vi "PID Autotuning.vi"(4 "autotune? (F)":bool, 5 "autotuning parameters":T2={"controller type"=1, "relay cycles"=3, "relay amplitude"=1.0, "control specification"=2, "PV noise level"=0.1} {"PV noise level" format="%.2f"; "control specification" items=["normal", "fast", "slow"]; "relay amplitude" format="%.2f"; "controller type" items=["PID", "PI", "P"]}, 6 "reinitialize? (F)":bool, 7 "output range":cluster{"output high":dbl, "output low":dbl}={"output high"=100.0, "output low"=-100.0} {"output low" format="%.2f"; "output high" format="%.2f"}, 8 "dt (s)":dbl=-1.0 format="%.3f", 9 "PID gains":T1={"proportional gain (Kc)"=1.0, "integral time (Ti, min)"=0.01, "derivative time (Td, min)"=0.0} {"derivative time (Td, min)" format="%.3f"; "integral time (Ti, min)" format="%.3f"; "proportional gain (Kc)" format="%.3f"}, 10 "process variable":dbl format="%.2f", 11 "setpoint":dbl format="%.2f") -> (0 "dt out (s)":dbl format="%.3f", 1 "PID gains out":T1={"proportional gain (Kc)"=1.0, "integral time (Ti, min)"=0.01, "derivative time (Td, min)"=0.0} {"derivative time (Td, min)" format="%.3f"; "integral time (Ti, min)" format="%.3f"; "proportional gain (Kc)" format="%.3f"}, 2 "tuning completed?":bool, 3 "output":dbl format="%.2f")   [LabVIEW 2017, in "NI_PID_autopid.lvlib"]
doc: "Includes the Autotuning Wizard in addition to the basic PID algorithm. You can use this VI instead of the PID VI, which implements a basic PID algorithm. Use the additional inputs and output of this VI to set autotuning parameters, invoke the Autotuning Wizard, and update the PID gains."
uses:
  <vilib>/addons/control/pid/NI_PID_autopid.lvlib
  <vilib>/addons/control/pid/NI_PID_pid.lvlib
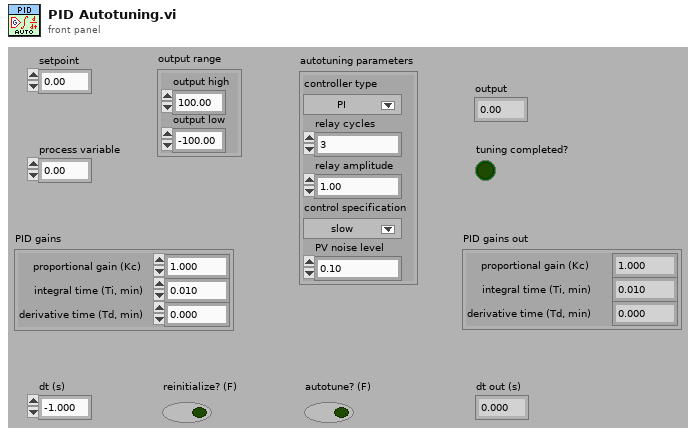
[diagram p1: front panel]
types:
  T1 = cluster{"proportional gain (Kc)":dbl, "integral time (Ti, min)":dbl, "derivative time (Td, min)":dbl}
  T2 = cluster{"controller type":u16, "relay cycles":i32, "relay amplitude":dbl, "control specification":u16, "PV noise level":dbl}
  T3 = enum16{"Normal", "Start", "Check params", "Check noise", "Start noise est.", "Re-estimate noise", "Begin autotune", "Autotuning", "New parameters", ""}
  T4 = cluster{"process variable":dbl, "setpoint out":dbl, "output":dbl}
  T5 = cluster{"Controller Type":u16, "# of cycles to avg":i32, "Relay amplitude":dbl, "Control design  ":u16, "Noise level":dbl}
  T6 = cluster{"Kc":dbl, "Ti (min)":dbl, "Td (min)":dbl}
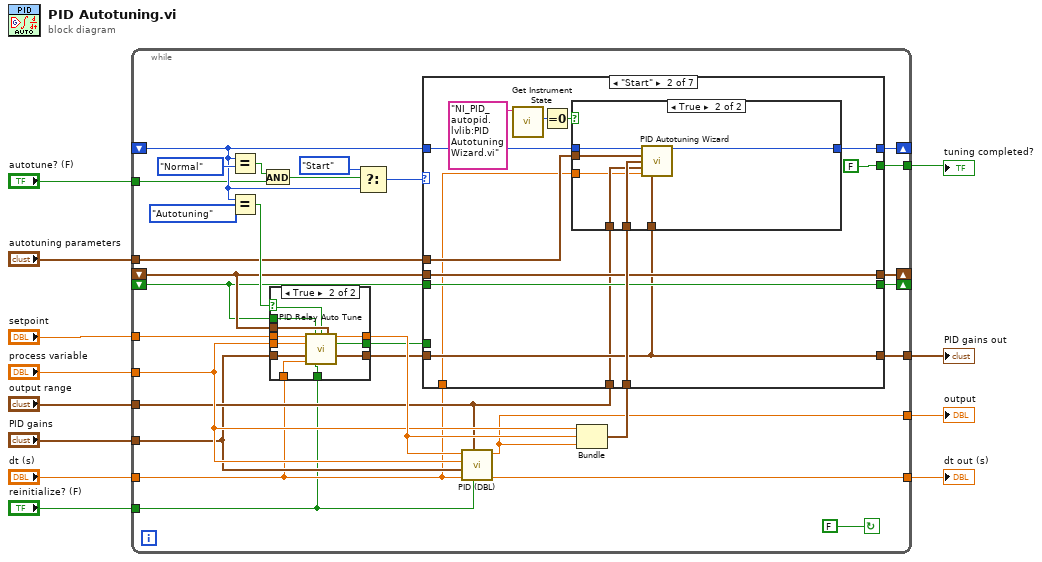
[diagram p0: block diagram]
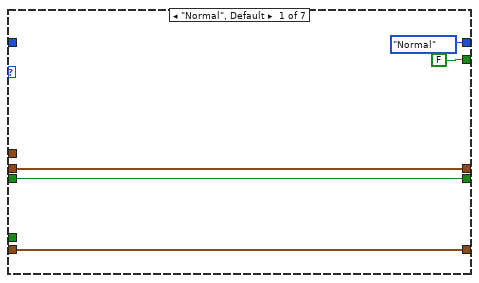
[diagram p2: hidden frame]
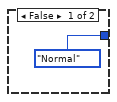
[diagram p3: hidden frame]
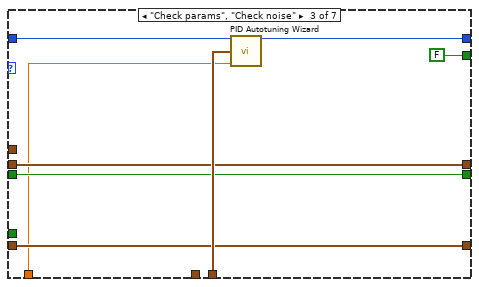
[diagram p4: hidden frame]
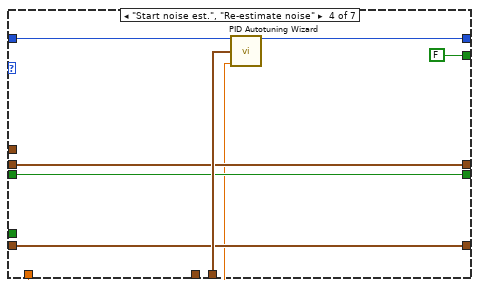
[diagram p5: hidden frame]
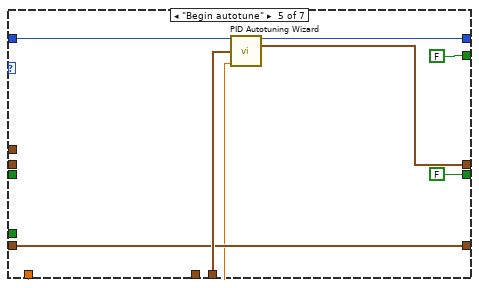
[diagram p6: hidden frame]
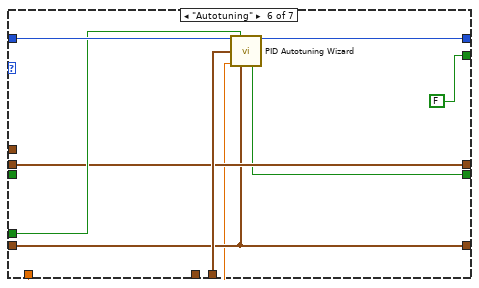
[diagram p7: hidden frame]
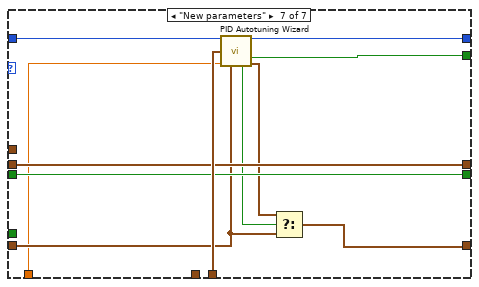
[diagram p8: hidden frame]
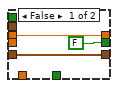
[diagram p9: hidden frame]
diagram:
  n1 = while {
    shift-left: _ -> [w33]
    shift-right: [w32] -> _
    shift-left: _ -> [w34]
    shift-right: [w35] -> _
    shift-left: _ -> [w25]
    shift-right: [w42] -> _
    tunnel: "setpoint" -> [w24]
    tunnel: "process variable" -> [w23]
    tunnel: "output range" -> [w22]
    tunnel: "PID gains" -> [w21]
    tunnel: "dt (s)" -> [w20]
    tunnel: "reinitialize? (F)" -> [w19]
    tunnel: "autotune? (F)" -> [w18]
    tunnel: "autotuning parameters" -> [w17]
    tunnel: [w16] -> w4
    tunnel: [w15] -> w3
    tunnel: [w14] -> w2
    tunnel: [w13] -> w1
    stop <- FALSE continue-if-true
    n2 = Equal?(x=w25, y=T3."Normal" ("states")) -> (x = y?=w31:bool)
    n3 = Equal?(x=w25, y=T3."Autotuning" ("states")) -> (x = y?=w40:bool)
    n4 = And(x=w31, y=w18) -> (x .and. y?=w39:bool)
    n5 = case shown="True" w40 {
      selector: w40 -> [_ w116]
      tunnel: [w115 w117] -> w41
      tunnel: w24 -> [w115 w124]
      tunnel: [w113 w120] -> w37
      tunnel: w21 -> [w113 w126]
      tunnel: w23 -> [_ w125]
      tunnel: [FALSE ("tuning status") w119] -> w36
      tunnel: w34 -> [_ w123]
      tunnel: w33 -> [_ w121]
      tunnel: w20 -> [_ w122]
      tunnel: w19 -> [_ w118]
      frame False {
      }
      frame True {
        n6 = call <vilib>:"PID Relay Auto Tune.VI"("Setpoint in"=w124, "Calculate Parameters"=w121, "Relay Setpoint"=w116, "autotuning parameters"=w123, "Process Variable"=w125, "PID gains"=w126, "dt (s)"=w122, "reinitialize? (F)"=w118) -> ("setpoint out"=w117:dbl, "tuning completed?"=w119:bool, "tuned PID gains"=w120:T1)  [unwired: 5 out]
      }
    }
    n7 = Select(t=T3."Start" ("states"), s=w39, f=w25) -> (s? t:f=w27:T3)
    n8 = call <vilib>:"PID (DBL).vi"("reinitialize? (F)"=w19, "output range"=w22, "dt (s)"=w20, "PID gains"=w21, "process variable"=w23, "setpoint"=w41) -> ("dt out (s)"=w15:dbl, "output"=w16:dbl)  [unwired: 1 in, 3 out]
    n9 = Bundle("process variable"=w23, "setpoint out"=w41, "output"=w16) -> (w38:T4)  [unwired: 1 out]
    n10 = case shown="\"Start\"" w27 {
      tunnel: [T3."Normal" ("states") w59 w74 w82 w90 w99 w111] -> w42
      tunnel: [FALSE FALSE FALSE FALSE FALSE FALSE w107] -> w13
      tunnel: w38 -> [_ w54 w73 w81 w89 w98 w110]
      tunnel: w25 -> [_ w55 w75 w83 w91 w100 w112]
      tunnel: w37 -> [w44 w51 w70 w78 w87 w94 w104]
      tunnel: w36 -> [_ _ _ _ _ w97 _]
      tunnel: [w46 w52 w72 w79 w88 w96 w109] -> w35
      tunnel: w34 -> [w46 w52 w72 w79 _ w96 w109]
      tunnel: [w45 w53 w71 w80 FALSE ("yes/no") w95 w108] -> w32
      tunnel: w33 -> [w45 w53 w71 w80 _ _ w108]
      tunnel: [w44 w51 w70 w78 w87 w94 w103] -> w14
      tunnel: w22 -> [_ w50 _ _ _ _ _]
      tunnel: w17 -> [_ w49 _ _ _ _ _]
      tunnel: w20 -> [_ w48 w69 w77 w85 w93 w102]
      frame "Normal", Default {
      }
      frame "Start" {
        n11 = call <vilib>:"Get Instrument State.vi"("VI name"="NI_PID_autopid.lvlib:PID Autotuning Wizard.vi") -> ("window state"=w57:enum32{"Closed", "Open", "Open and Active"})  [unwired: 1 in, 9 out]
        n12 = Equal To 0?(x=w57) -> (x = 0?=w56:bool)
        n13 = case shown="True" w56 {
          tunnel: [T3."Normal" ("states") w67] -> w59
          tunnel: w55 -> [_ w68]
          tunnel: w54 -> [_ w66]
          tunnel: w49 -> [_ w65]
          tunnel: w51 -> [_ w64]
          tunnel: w50 -> [_ w63]
          tunnel: w48 -> [_ w62]
          frame False {
          }
          frame True {
            n14 = call <vilib>:"PID Autotuning Wizard.vi"("states"=w68, "autotuning parameters"=w65, "Control Signals"=w66, "output range"=w63, "dt (s)"=w62, "new PID parameters input"=w64) -> ("state out"=w67:T3)  [unwired: 1 in, 8 out]
          }
        }
      }
      frame "Check params", "Check noise" {
        n15 = call <vilib>:"PID Autotuning Wizard.vi"("states"=w75, "Control Signals"=w73, "dt (s)"=w69) -> ("state out"=w74:T3)  [unwired: 4 in, 8 out]
      }
      frame "Start noise est.", "Re-estimate noise" {
        n16 = call <vilib>:"PID Autotuning Wizard.vi"("states"=w83, "Control Signals"=w81, "dt (s)"=w77) -> ("state out"=w82:T3)  [unwired: 4 in, 8 out]
      }
      frame "Begin autotune" {
        n17 = call <vilib>:"PID Autotuning Wizard.vi"("states"=w91, "Control Signals"=w89, "dt (s)"=w85) -> ("state out"=w90:T3, "autotuning parameters out"=w88:T5)  [unwired: 4 in, 7 out]
      }
      frame "Autotuning" {
        n18 = call <vilib>:"PID Autotuning Wizard.vi"("states"=w100, "tuning completed?"=w97, "Control Signals"=w98, "dt (s)"=w93, "new PID parameters input"=w94) -> ("state out"=w99:T3, "yes/no out"=w95:bool)  [unwired: 2 in, 7 out]
      }
      frame "New parameters" {
        n19 = call <vilib>:"PID Autotuning Wizard.vi"("states"=w112, "Control Signals"=w110, "dt (s)"=w102, "new PID parameters input"=w104) -> ("state out"=w111:T3, "complete?"=w107:bool, "yes/no out"=w106:bool, "new PID parameters out"=w105:T6)  [unwired: 3 in, 5 out]
        n20 = Select(t=w105, s=w106, f=w104) -> (s? t:f=w103:T1)
      }
    }
  }
  "output" <- w4
  "dt out (s)" <- w3
  "PID gains out" <- w2
  "tuning completed?" <- w1
